vi "Header or Footer Same Line.vi"(1 "Header Footer [ ] IN":T1) -> (0 "Header Footer [ ] OUT":T1)   [LabVIEW 2012]
doc: "Version 1.0\nDeveloped by Jean-Marc Simard\nCopyright © 2010, Exaprom Inc.\nAll rights reserved.\nLicense: BSD"
uses:
  Controls/Header Footer [ ].ctl
  Controls/Header Footer cluster.ctl
  Controls/Header Footer Type.ctl
  Controls/Header footer horiz alignment.ctl
  Controls/Cell Vertical alignment.ctl
  Controls/Page number.ctl
  Controls/Font cluster.ctl
  Controls/Font size.ctl
  Controls/Font color.ctl
  C:/Users/MaxCorp/Documents/TopPerm - Base/DLL/itextsharp.dll
  DLL/itextsharp.dll
  Controls/Header Footer Line.ctl
panel:
  # "X"
  # "Y"
  # "X"
  # "Y"
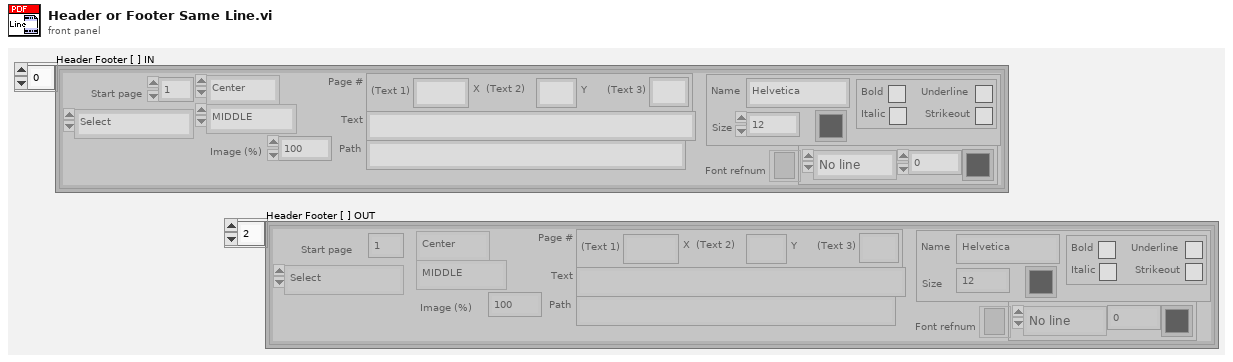
[diagram p1: front panel]
types:
  T1 = typedef "Header Footer [ ].ctl" = T2[]
  T2 = typedef "Header Footer cluster.ctl" = cluster{"Start page":i32, "Type":T3, "Alignment":T4, "Vertical Alignement":T5, "Image (%)":sgl, "Page #":T6, "Text":string, "Path":string, "Font":T7, "Font refnum":refnum<k24>, "Line":cluster{"Line":T10, "Thickness (points)":sgl, "Colour":T9}}
  T3 = typedef "Header Footer Type.ctl" = enum16{"Select", "Text", "Text + hyperlink", "Page number", "Image", "Image + hyperlink"}
  T4 = typedef "Header footer horiz alignment.ctl" = enum16{"Left", "Center", "Right"}
  T5 = typedef "Cell Vertical alignment.ctl" = enum16{"TOP", "MIDDLE", "BOTTOM"}
  T6 = typedef "Page number.ctl" = cluster{"Text 1":string, "Text 2":string, "Text 3":string}
  T7 = typedef "Font cluster.ctl" = cluster{"Name":string, "Size":T8, "Color":T9, "Style":cluster{"Bold":bool, "Italic":bool, "Underline":bool, "Strikeout":bool}}
  T8 = typedef "Font size.ctl" = sgl
  T9 = typedef "Font color.ctl" = u32
  T10 = typedef "Header Footer Line.ctl" = enum16{"No line", "Horizontal line"}
  T11 = cluster{"Line":T10, "Thickness (points)":sgl, "Colour":T9}
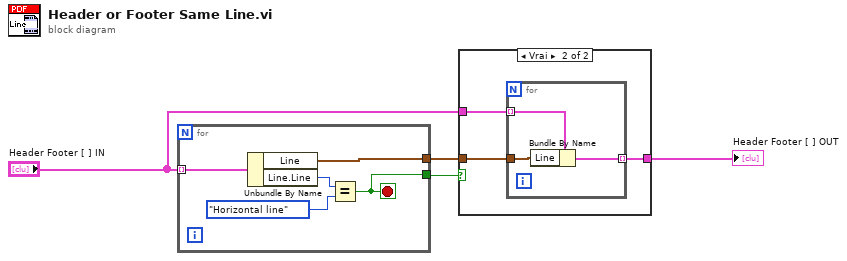
[diagram p0: block diagram]
diagram:
  n1 = for {
    tunnel: "Header Footer [ ] IN" -> [w6] mode=indexing
    tunnel: [w7] -> w1
    tunnel: [w5] -> w3
    stop <- w7 stop-if-true
    n2 = Unbundle By Name(w6) -> ("Line"=w5:T11, "Line.Line"=w9:T10)
    n3 = Equal?(x=w9, y=Header_Footer_Line."Horizontal line") -> (x = y?=w7:bool)
  }
  n4 = case shown="Vrai" w1 {
    tunnel: "Header Footer [ ] IN" -> [w10 w13]
    tunnel: w3 -> [_ w12]
    tunnel: [w10 w11] -> w2
    frame False {
    }
    frame True {
      n5 = for {
        tunnel: w13 -> [w16] mode=indexing
        tunnel: w12 -> [w15]
        tunnel: [w14] -> w11 mode=indexing
        n6 = Bundle By Name(cluster=w16, "Line"=w15) -> (w14:T2)
      }
    }
  }
  "Header Footer [ ] OUT" <- w2
